vi "fib.vi"() -> ()   [LabVIEW 2017]
panel:
  out "斐波那契":i64
  in  "第":i32
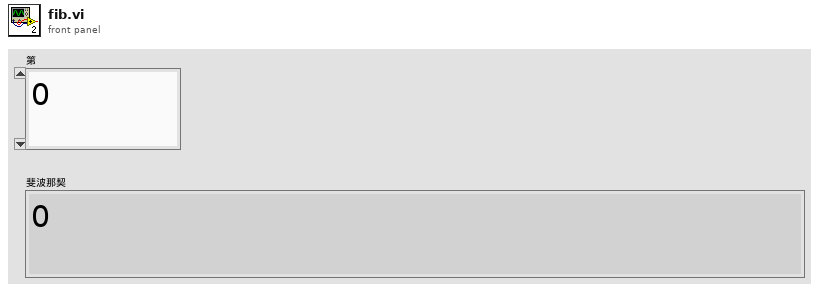
[diagram p1: front panel]
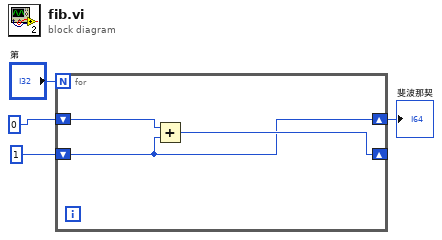
[diagram p0: block diagram]
diagram:
  n1 = for {
    N: "第" -> [_]
    shift-right: [w5] -> w1
    shift-left: i64 0 -> [w7]
    shift-right: [w6] -> _
    shift-left: i64 1 -> [w5]
    n2 = Add(x=w7, y=w5) -> (x+y=w6:i64)
  }
  "斐波那契" <- w1
